vi "LINC Push.vi"(8 "error in (no error)":errorcluster, 11 "parameters":T1) -> (0 "error out":errorcluster)   [LabVIEW 2018, in "STEPkgDriver_LINC.lvlib"]
uses:
  STEPkgDriver_LINC.lvlib
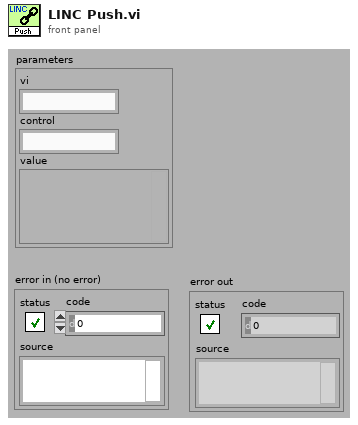
[diagram p1: front panel]
types:
  T1 = cluster{"vi":string, "control":string, "value":variant}
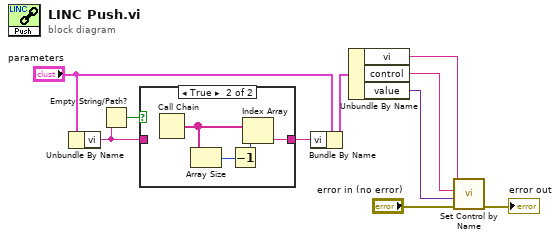
[diagram p0: block diagram]
diagram:
  n1 = Unbundle By Name("parameters") -> ("vi"=w4:string)
  n2 = Empty String/Path?(string/path=w4) -> (empty?=w3:bool)
  n3 = case shown="True" w3 {
    tunnel: [w11 w15] -> w5
    tunnel: w4 -> [w11 _]
    frame False {
    }
    frame True {
      n4 = Call Chain() -> (call chain=w14:string[])
      n5 = Array Size(array=w14) -> (size(s)=w13:i32)
      n6 = Decrement(x=w13) -> (x-1=w12:i32)
      n7 = Index Array(array=w14, index=w12) -> (element=w15:string)
    }
  }
  n8 = Bundle By Name(cluster="parameters", "vi"=w5) -> (w6:T1)
  n9 = Unbundle By Name(w6) -> ("vi"=w7:string, "control"=w8:string, "value"=w9:variant)
  n10 = call "Set Control by Name.vi"("error in (no error)"="error in (no error)", "value"=w9, "control name"=w8, "vi name"=w7) -> ("error out"=→"error out":errorcluster)  [unwired: 7 in]
